vi "WiiMote Interface.vi"() -> ()   [LabVIEW 2013]
doc: "Uses the General Histogram VI to implement a running histogram.\n\nThis example generates continuous Gaussian noise, computes the histogram of the noise, and adds the new histogram to the sum of all the previous histograms.\n\nIn addition to computing the histogram, the General Histogram VI also computes the number of points that are outside all bins. This example keeps a running total of this quantity. The bins of the histogram span three standard deviations of the noise level.\n\nThe histogram plot should begin to resemble a Gaussian curve as more points are added to the histogram. The units of the histogram display are % of total points. \n\nNote: You must have the LabVIEW Full or Professional Development Systems to run this example. Also note that there is now a Point by Point function palette which provides an easier way to implement a running histogram. See the example Moving Histogram PtByPt.vi."
uses:
  D:/Users/jjensen/Documents/Lab Book/embeddedLab/exercises/LabVIEW/WiiMote/Dependencies/WiimoteLib.dll
  Dependencies/WiimoteLib.dll
  <vilib>/Analysis/coordinate.llb/Angle Units.ctl
  <vilib>/Analysis/coordinate.llb/Wrap Angle (array).vi
  <vilib>/imath/engines/lvmath2/RunTimeEngine/NodeEndStatement/NIMS_NodeEndStatement_Output.vi
  <instcachedir>/0/NIMS_NodeEndStatement_Output_53EC0D466D134D7ABD903AC30B43404B.lvgen/NIMS_NodeEndStatement_Output_53EC0D466D134D7ABD903AC30B43404B_010.vi
  <instcachedir>/0/NIMS_NodeEndStatement_Output_53EC0D466D134D7ABD903AC30B43404B.lvgen/NIMS_NodeEndStatement_Output_53EC0D466D134D7ABD903AC30B43404B_011.vi
  <vilib>/imath/engines/lvmath2/RunTimeEngine/ErrorHandling/NIMS_Finalize Error.vi
  <vilib>/Analysis/NI_AAL_Angle.lvlib
panel:
  in  "calibration (raw)":cluster{"bias":i32, "sensitivity":i32}={"bias"=0, "sensitivity"=1}
  out "Orientation (calibrated)":cluster{"Angle Out[0]":dbl, "Angle Out[1]":dbl}(graph)
  out "magnitude (g)":dbl
  out "Acceleration (calibrated)":cluster{"a[0]":i16, "a[1]":i16, "a[2]":i16}(graph)
  out "Acceleration (uncalibrated)":cluster{"X":sgl, "Y":sgl, "Z":sgl}(graph)
  in  "HID Transmit":u8=82 format="%02x"
  in  "measure sensitivity":bool
  in  "measure bias":bool caption="Record x-axis d0"
  in  "Payload":u8 format="%02x"
  in  "Report ID":u8 format="%02x"
  in  "Transmit":bool
  in  "stop":bool
  # "x"
  # "x"
  # "y"
  # "y"
  # "z"
  # "z"
  # "Calibration"
  # "Transmission"
  # "Measure"
  # "roll"
  # "pitch"
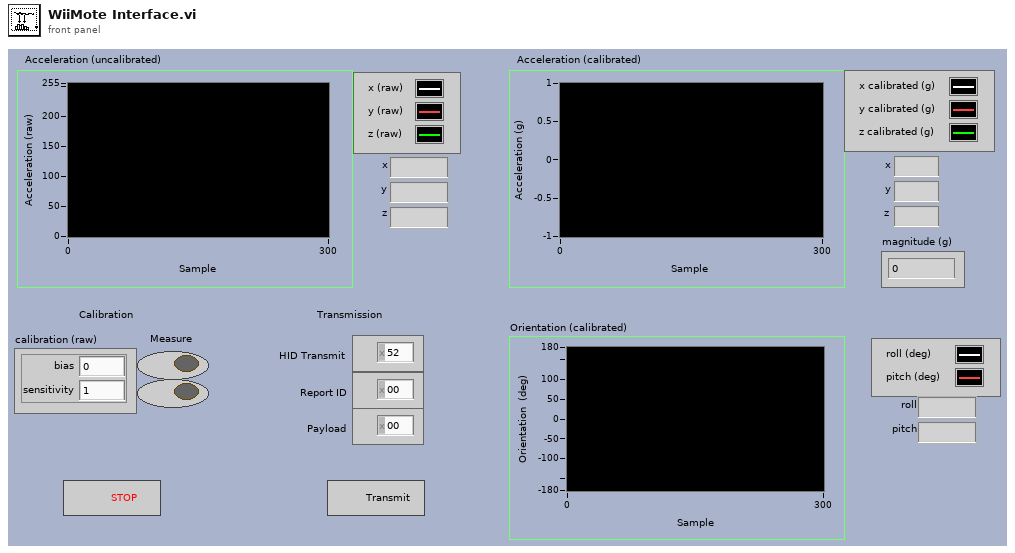
[diagram p1: front panel]
types:
  T1 = typedef "WiiMote State.ctl" = cluster{"X":sgl, "Y":sgl, "Z":sgl, "A":bool, "B":bool, "Down":bool, "Home":bool, "Left":bool, "Minus":bool, "One":bool, "Plus":bool, "Right":bool, "Two":bool, "Up":bool, "error out":errorcluster}
  T2 = typedef "NI_AAL_Angle.lvlib/Angle Units.ctl" = i32
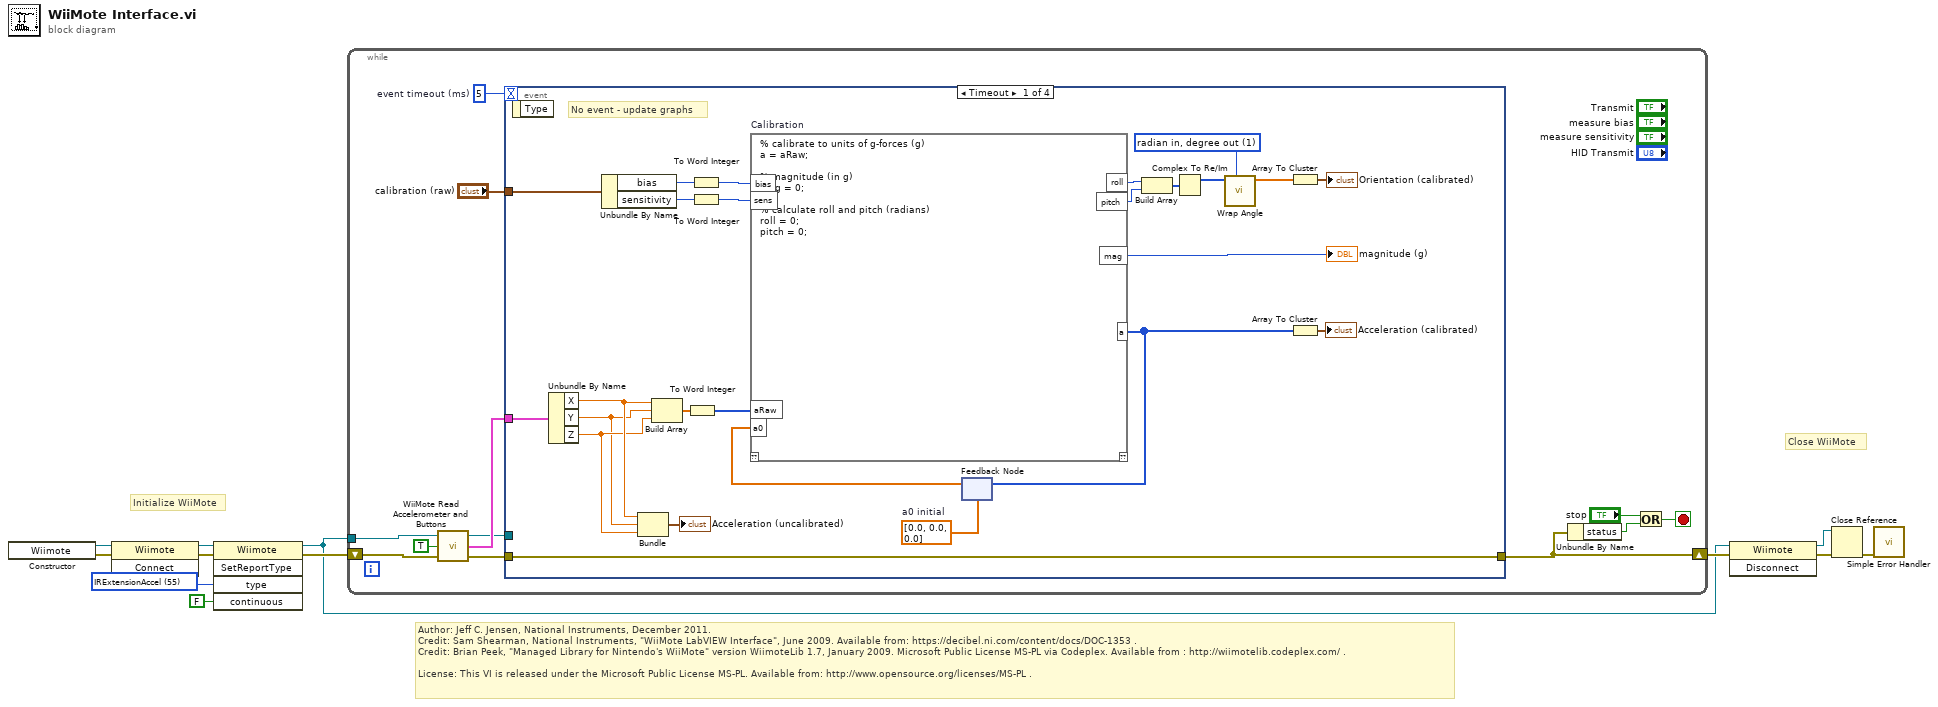
[diagram p0: block diagram]
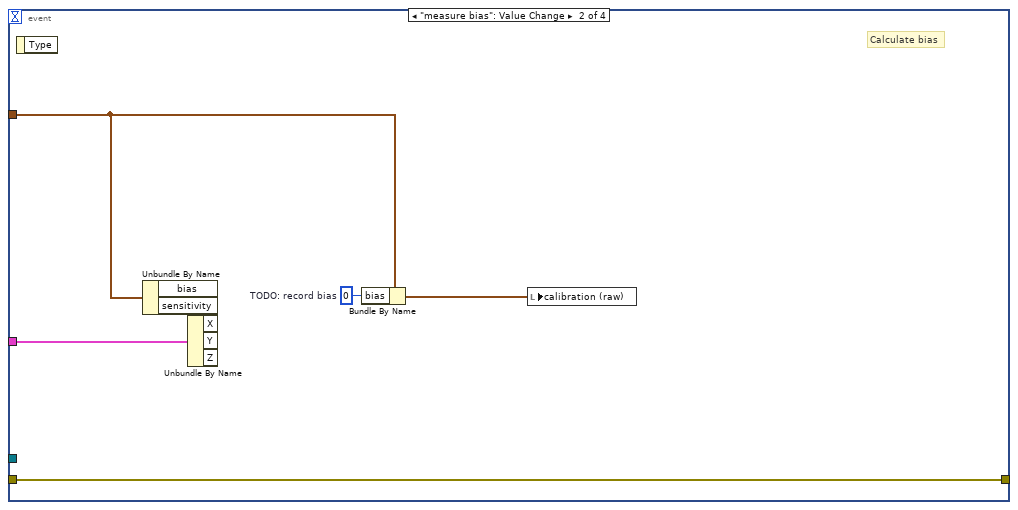
[diagram p2: hidden frame]
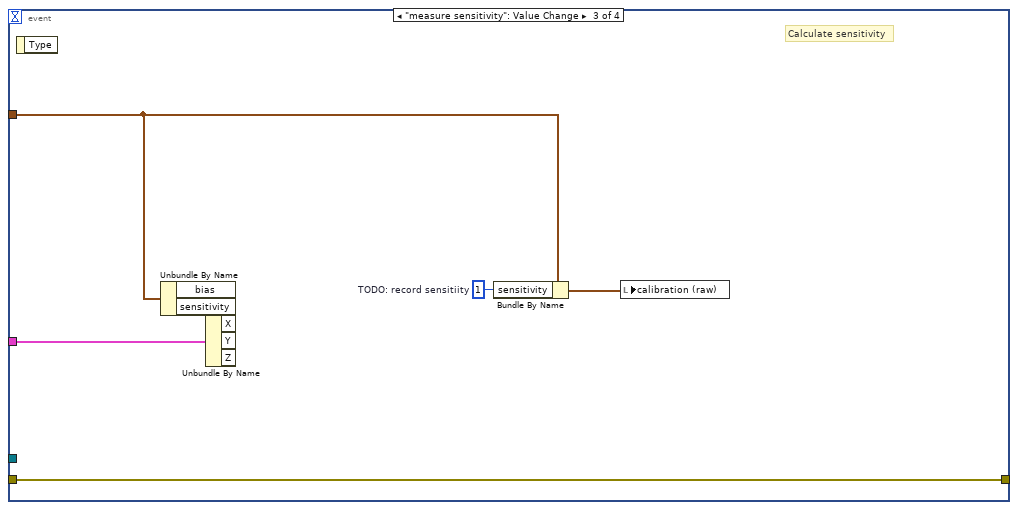
[diagram p3: hidden frame]
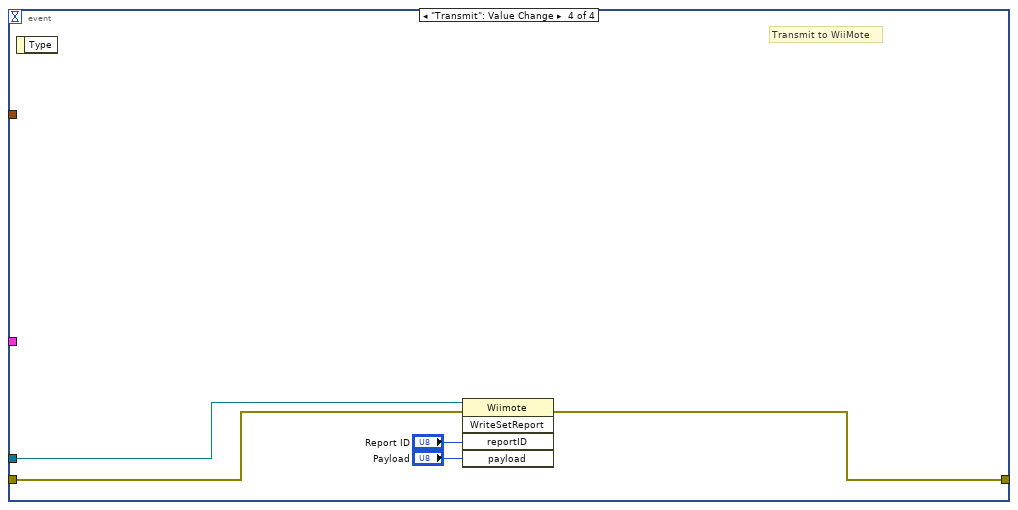
[diagram p4: hidden frame]
diagram:
  w10 = u8 55 items=["Status"=32, "ReadData"=33, "OutputReportAck"=34, "Buttons"=48, "ButtonsAccel"=49, "IRAccel"=51, "ButtonsExtension"=52, "ExtensionAccel"=53, "IRExtensionAccel"=55] ("type")
  # "Author: Jeff C. Jensen, National Instruments, December 2011.\nCredit: Sam Shearman, National Instruments, \"WiiMote LabVIEW Interface\", June 2009. Available from: https://decibel.ni.com/content/docs/DOC-1353 .\nCredit: Brian Peek, \"Managed Library for Nintendo's WiiMote\" version WiimoteLib 1.7, January 2009. Microsoft Public License MS-PL via Codeplex. Available from : http://wiimotelib.codeplex.com/ .\n\nLicense: This VI is released under the Microsoft Public License MS-PL. Available from: http://www.opensource.org/licenses/MS-PL ."
  # "Close WiiMote"
  # "Initialize WiiMote"
  n1 = constructor class="Wiimote"() -> (reference out=w11:refnum<k24>, error out=w12:errorcluster)  [unwired: 3 in, 1 out]
  n2 = invoke class="Wiimote" method="Connect"(reference=w11, error in=w12) -> (reference out=w1:refnum<k24>, error out=w8:errorcluster)  [unwired: 1 in, 1 out]
  n3 = invoke class="Wiimote" method="SetReportType"(reference=w1, error in=w8, "type"=w10, "continuous"=FALSE) -> (reference out=w3:refnum<k24>, error out=w7:errorcluster)  [unwired: 1 in, 3 out]
  n4 = while {
    tunnel: w3 -> [w23]
    shift-right: [w17] -> w9
    shift-left: w7 -> [w22]
    stop <- w24 stop-if-true
    w21 = 5  # event timeout (ms)
    n5 = call "WiiMote Read Accelerometer and Buttons.vi"("error in"=w22, "read raw values"=TRUE, "Wiimote"=w23) -> ("error out"=w19:errorcluster, "Wiimote State"=w20:T1, "reference out"=w18:refnum<k24>)
    n6 = event shown="[0] Timeout" {
      selector: _ -> [_ _ _ _]
      dyn-events: _ -> [_ _ _ _]
      timeout: w21 -> [_ _ _ _]
      tunnel: w20 -> [w49 w92 w98 _]
      tunnel: w19 -> [w48 w93 w97 w101]
      tunnel: w18 -> [_ _ _ w100]
      tunnel: [w48 w93 w97 w99] -> w17
      tunnel: "calibration (raw)" -> [w44 w90 w96 _]
      event Timeout {
        w26 = T2 1 items=["radian in, radian out", "radian in, degree out", "degree in, degree out", "degree in, radian out"] ("angle units")
        w36 = dbl[] [0.0, 0.0, 0.0]  # a0 initial
        # "No event - update graphs"
        n7 = event-data() -> ()  [unwired: 1 in, 1 out]
        n8 = Unbundle By Name(w49) -> ("X"=w43:sgl, "Y"=w41:sgl, "Z"=w42:sgl)
        n9 = Unbundle By Name(w44) -> ("bias"=w46:i32, "sensitivity"=w45:i32)
        n10 = Bundle("X"=w43, "Y"=w41, "Z"=w42) -> (→"Acceleration (uncalibrated)":cluster{"X":sgl, "Y":sgl, "Z":sgl})  [unwired: 1 in]
        n11 = Build Array(w43, w41, w42) -> (w40:sgl[])
        n12 = To Word Integer(number=w40) -> (16bit integer=w37:i16[])
        n13 = To Word Integer(number=w46) -> (16bit integer=w39:i16)
        n14 = To Word Integer(number=w45) -> (16bit integer=w38:i16)
        n15 = feedback #1(w36) -> (w32:dbl[])
        n16 = mathscript code="% calibrate to units of g-forces (g)\na = aRaw;\n\n% magnitude (in g)\nmag = 0;\n\n% calculate roll and pitch (radians)\nroll = 0;\npitch = 0;" "Calibration"("bias"=w39, "sens"=w38, "aRaw"=w37, "a0"=w32) -> ("mag"=→"magnitude (g)":i32, "a"=w33:i16[], "roll"=w29:i32, "pitch"=w28:i32)  [unwired: 1 in, 1 out]
        n17 = feedback-in #1(w33) -> ()
        n18 = Build Array(w29, w28) -> (w35:i32[])
        n19 = Complex To Re/Im(x + iy=w35) -> (x=w27:i32[])  [unwired: 1 out]
        n20 = call-poly <vilib>:"Wrap Angle.vi"("angle units"=w26, "Angle In"=w27) -> ("Angle Out"=w25:dbl[])  [unwired: 8 in, 1 out]
        n21 = Array To Cluster(array=w25) -> (cluster=→"Orientation (calibrated)":cluster{"Angle Out[0]":dbl, "Angle Out[1]":dbl})
        n22 = Array To Cluster(array=w33) -> (cluster=→"Acceleration (calibrated)":cluster{"a[0]":i16, "a[1]":i16, "a[2]":i16})
      }
      event "measure bias": Value Change {
        w89 = 0  # TODO: record bias
        # "Calculate bias"
        n23 = event-data() -> ()  [unwired: 1 in, 1 out]
        n24 = Unbundle By Name(w90) -> ()  [unwired: 2 out]
        n25 = Unbundle By Name(w92) -> ()  [unwired: 3 out]
        n26 = Bundle By Name(cluster=w90, "bias"=w89) -> (w91:cluster{"bias":i32, "sensitivity":i32})
        n27 = local write "calibration (raw)"(w91) -> ()
      }
      event "measure sensitivity": Value Change {
        w94 = 1  # TODO: record sensitiity
        # "Calculate sensitivity"
        n28 = event-data() -> ()  [unwired: 1 in, 1 out]
        n29 = Unbundle By Name(w96) -> ()  [unwired: 2 out]
        n30 = Unbundle By Name(w98) -> ()  [unwired: 3 out]
        n31 = Bundle By Name(cluster=w96, "sensitivity"=w94) -> (w95:cluster{"bias":i32, "sensitivity":i32})
        n32 = local write "calibration (raw)"(w95) -> ()
      }
      event "Transmit": Value Change {
        # "Transmit to WiiMote"
        n33 = event-data() -> ()  [unwired: 1 in, 1 out]
        n34 = invoke class="Wiimote" method="WriteSetReport"(reference=w100, error in=w101, "reportID"="Report ID", "payload"="Payload") -> (error out=w99:errorcluster)  [unwired: 1 in, 4 out]
      }
    }
    n35 = Unbundle By Name(w17) -> ("status"=w15:bool)
    n36 = Or(x="stop", y=w15) -> (x .or. y?=w24:bool)
  }
  n37 = invoke class="Wiimote" method="Disconnect"(reference=w3, error in=w9) -> (reference out=w6:refnum<k24>, error out=w5:errorcluster)  [unwired: 1 in, 1 out]
  n38 = Close Reference(reference=w6, error in (no error)=w5) -> (error out=w4:errorcluster)
  n39 = call <vilib>:"Simple Error Handler.vi"("error in (no error)"=w4) -> ()  [unwired: 4 in, 5 out]
